vi "Determine Warning.vi"() -> ()   [LabVIEW 2014]
panel:
  out "Warning":bool
  out "Warning Tex":string
  in  "Min Temp":dbl
  in  "Max temp":dbl
  in  "Current Temp":dbl
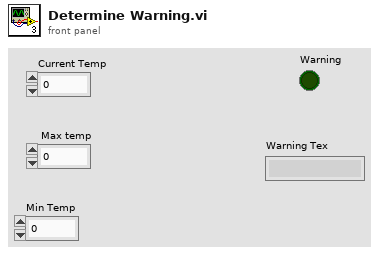
[diagram p1: front panel]
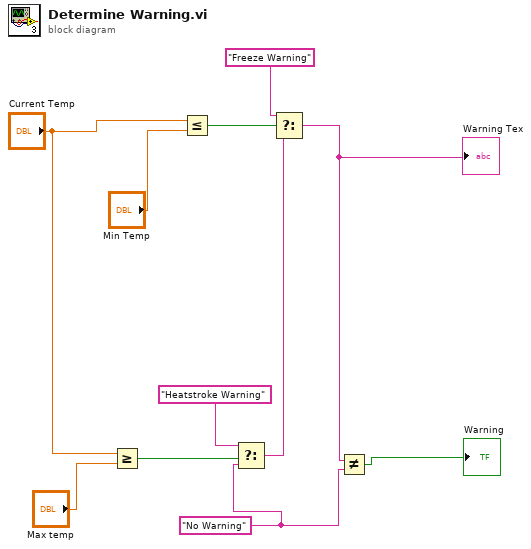
[diagram p0: block diagram]
diagram:
  w5 = "No Warning"
  n1 = Greater Or Equal?(x="Current Temp", y="Max temp") -> (x >= y?=w7:bool)
  n2 = Less Or Equal?(x="Current Temp", y="Min Temp") -> (x <= y?=w3:bool)
  n3 = Select(t="Heatstroke Warning", s=w7, f=w5) -> (s? t:f=w4:string)
  n4 = Select(t="Freeze Warning", s=w3, f=w4) -> (s? t:f=w1:string)
  "Warning Tex" <- w1
  n5 = Not Equal?(x=w1, y=w5) -> (x != y?=→"Warning":bool)
